vi "cDAQ Open ADC.vi"(8 "error in":errorcluster, 10 "Reset (False)":bool, 11 "cdaq session in":T1={"mclk [Hz]"=12800000.0, "ADC task"="", "mclk reference"="", "fs [Hz]"=50000.0, "queue adc cmd"=refnum, "queue adc data"=refnum, "adc proc ref"=refnum, "channels"=[], "last channels"=[], "timeout"=timestamp(0 s since 1904-01-01), "N"=1000, "mclk mode"=enum."Free running", "ext mclk source"=""} {"last channels"."Channel id" min=0 step=1; "channels"."Channel id" min=0 step=1}) -> (0 "error out":errorcluster, 2 "channel idns":string[](array[string]), 3 "cdaq session out":T1={"mclk [Hz]"=12800000.0, "ADC task"="", "mclk reference"="", "fs [Hz]"=50000.0, "queue adc cmd"=refnum, "queue adc data"=refnum, "adc proc ref"=refnum, "channels"=[], "last channels"=[], "timeout"=timestamp(0 s since 1904-01-01), "N"=1000, "mclk mode"=enum."Free running", "ext mclk source"=""} {"last channels"."Channel id" min=0 step=1; "channels"."Channel id" min=0 step=1})   [LabVIEW 2020]
uses:
  cDAQ Session.ctl
  low_level_old/cdaq_anal_adc_command.ctl
  low_level_old/cdaq_anal_adc_data.ctl
  cDAQ Virtual Channel.ctl
  cDAQ Master Clock Mode.ctl
  <vilib>/Utility/error.llb/Error Cluster From Error Code.vi
  <vilib>/DAQmx/create/channels.llb/DAQmx Create Channel (AI-Voltage-Basic).vi
  <vilib>/DAQmx/configure/timing.llb/DAQmx Timing (Sample Clock).vi
  <vilib>/ErrorRing/Error Ring.xnode
  <resource>/objmgr/daqmx.rc
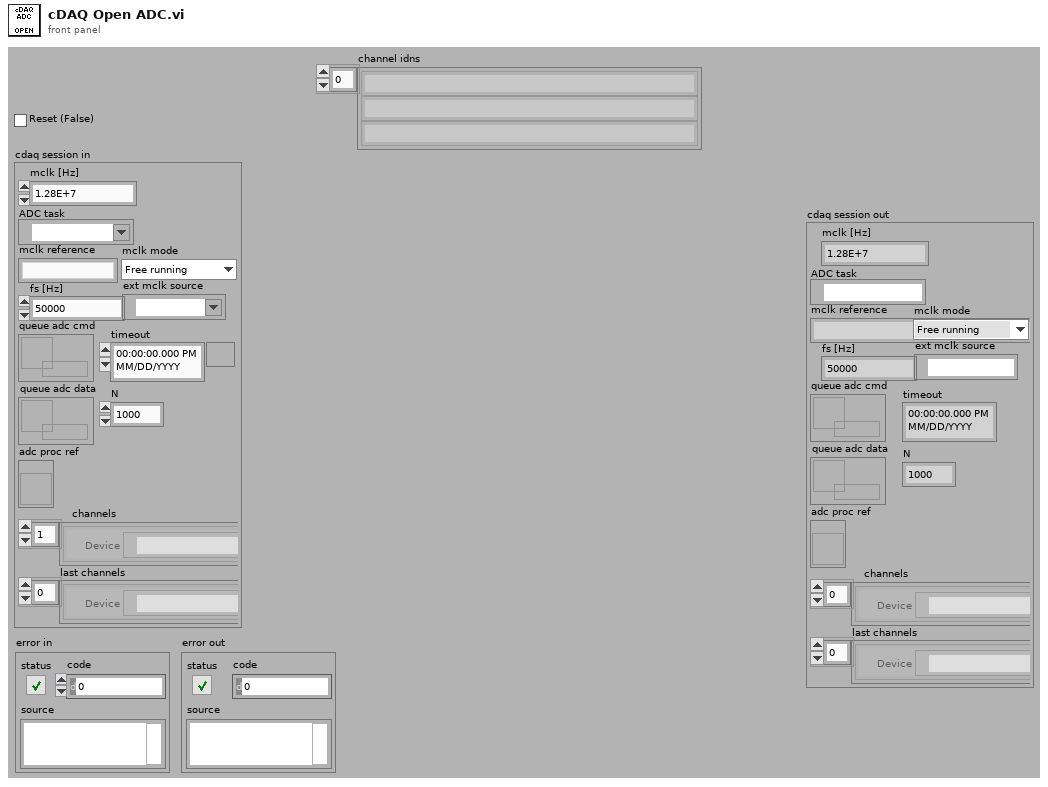
[diagram p1: front panel]
types:
  T1 = typedef "cDAQ Session.ctl" = cluster{"mclk [Hz]":dbl, "ADC task":refnum<k21>, "mclk reference":string, "fs [Hz]":dbl, "queue adc cmd":refnum<queue>, "queue adc data":refnum<queue>, "adc proc ref":refnum<vi>, "channels":T2[], "last channels":T2[], "timeout":timestamp, "N":i32, "mclk mode":T3, "ext mclk source":tag}
  T2 = typedef "cDAQ Virtual Channel.ctl" = cluster{"Device":tag, "Channel id":i32, "btn clr":bool, "btn up":bool, "btn down":bool}
  T3 = typedef "cDAQ Master Clock Mode.ctl" = enum16{"Free running", "Export master clock", "Import master clock"}
  T4 = typedef "cdaq_anal_adc_data.ctl" = cluster{"wave":dbl[][], "timestamp [s]":dbl, "abs timestamp":timestamp, "Aborted":bool}
  T5 = typedef "cdaq_anal_adc_command.ctl" = cluster{"sample to get":i32, "stop":bool, "abort":bool}
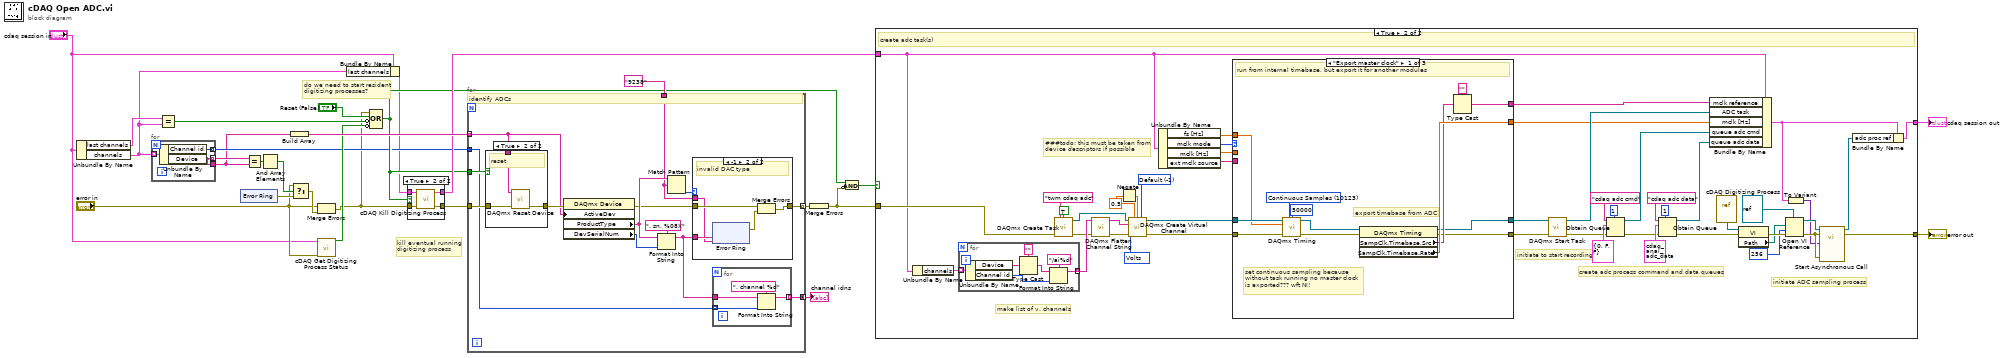
[diagram p0: block diagram]
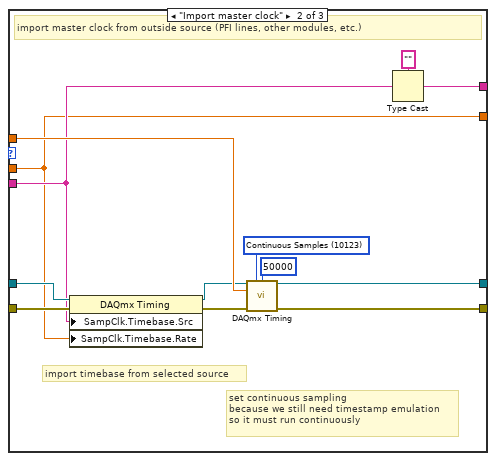
[diagram p4: hidden frame]
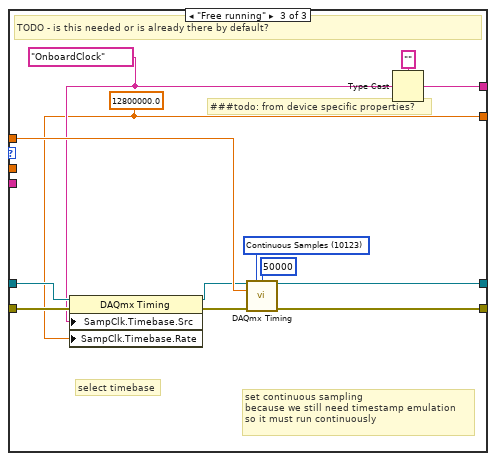
[diagram p5: hidden frame]
diagram:
  # "do we need to start resident\ndigitizing processes?"
  # "kill eventual running\ndigitizing process"
  n1 = Unbundle By Name("cdaq session in") -> ("last channels"=w18:T2[], "channels"=w2:T2[])
  n2 = for {
    tunnel: w2 -> [w30] mode=indexing
    tunnel: [w29] -> w24 mode=indexing
    tunnel: [w29] -> w5
    tunnel: [w28] -> w6 mode=indexing
    n3 = Unbundle By Name(w30) -> ("Channel id"=w28:i32, "Device"=w29:tag)
  }
  n4 = Equal?(x=w18, y=w2) -> (x = y?=w15:bool)
  n5 = xnode "Error Ring"() -> ("error out"=w21:errorcluster)
  n6 = Equal?(x=w24, y=w5) -> (x = y?=w23:bool[])
  n7 = And Array Elements(Boolean array=w23) -> (logical AND=w22:bool)
  n8 = Build Array(w5) -> (w19:tag[])
  n9 = Select(t="error in", s=w22, f=w21) -> (s? t:f=w20:errorcluster)
  n10 = call "cDAQ Get Digitizing Process Status.vi"("error in"="error in", "cdaq session"="cdaq session in") -> ("is running"=w14:bool)  [unwired: 7 in, 2 out]
  n11 = Merge Errors("error in", w20) -> (w4:errorcluster)
  n12 = Bundle By Name(cluster="cdaq session in", "last channels"=w2) -> (w3:T1)
  n13 = Compound Arithmetic op=OR(w4, "Reset (False)", invert w15, invert w14) -> (w9:bool)
  n14 = case shown="True" w9 {
    tunnel: w4 -> [w32 w36]
    tunnel: [w32 w35] -> w11
    tunnel: w3 -> [w31 w34]
    tunnel: [w31 w33] -> w10
    frame False {
    }
    frame True {
      n15 = call "cDAQ Kill Digitizing Process.vi"("error in"=w36, "cdaq session in"=w34) -> ("error out"=w35:errorcluster, "cdaq session out"=w33:T1)  [unwired: 8 in]
    }
  }
  n16 = for {
    tunnel: w19 -> [w49] mode=indexing
    tunnel: w11 -> [w43]
    tunnel: "9238" -> [w41]
    tunnel: [w42] -> w27 mode=indexing
    tunnel: w9 -> [w40]
    tunnel: w6 -> [w38]
    tunnel: [w37] -> w12 mode=concatenating
    # "identify ADCs"
    n17 = case shown="True" w40 {
      tunnel: [w55 w58] -> w50
      tunnel: w49 -> [_ w57]
      tunnel: w43 -> [w55 w56]
      frame False {
      }
      frame True {
        # "reset"
        n18 = call <vilib>:"DAQmx Reset Device.vi"("device in"=w57, "error in"=w56) -> ("error out"=w58:errorcluster)  [unwired: 13 in]
      }
    }
    n19 = property class="DAQmx Device"(error in=w50, "ActiveDev"=w49) -> (error out=w44:errorcluster, "ProductType"=w46:string, "DevSerialNum"=w48:u32)  [unwired: 1 in, 1 out]
    n20 = Format Into String(format string=", sn. %08X", initial string=w46, w48) -> (resulting string=w39:string)  [unwired: 1 in, 1 out]
    n21 = Match Pattern(string=w46, regular expression=w41) -> (offset past match=w45:i32)  [unwired: 1 in, 3 out]
    n22 = case shown="-1" w45 {
      tunnel: w44 -> [w59 w64]
      tunnel: w39 -> [_ w61]
      tunnel: [w59 w62] -> w42
      tunnel: w41 -> [_ w60]
      frame Default {
      }
      frame -1 {
        # "invalid DAC type"
        n23 = xnode "Error Ring"("parameter 0"=w61, "parameter 1"=w60) -> ("error out"=w63:errorcluster)
        n24 = Merge Errors(w64, w63) -> (w62:errorcluster)
      }
    }
    n25 = for {
      tunnel: w39 -> [w54]
      tunnel: w38 -> [w52] mode=indexing
      tunnel: [w51] -> w37 mode=indexing
      n26 = Format Into String(format string=", channel %d", initial string=w54, w52) -> (resulting string=w51:string)  [unwired: 1 in, 1 out]
    }
  }
  "channel idns" <- w12
  n27 = Merge Errors(w27) -> (w7:errorcluster)
  n28 = Compound Arithmetic op=AND(w9, invert w7) -> (w8:bool)
  n29 = case shown="True" w8 {
    tunnel: w10 -> [w74 w87]
    tunnel: [w73 w92] -> w26
    tunnel: [w74 w89] -> w25
    tunnel: w7 -> [w73 w88]
    frame False {
    }
    frame True {
      w113 = 0.5 ("maximum value")
      w122 = -1 items=["Default"=-1, "RSE"=10083, "Differential"=10106, "Pseudodifferential"=12529] ("output terminal configuration")
      w120 = 10348 items=["Volts"=10348, "From Custom Scale"=10065] ("units")
      # "###todo: this must be taken from\ndevice descriptors if possible"
      # "make list of v. channels"
      # "initiate ADC sampling process"
      # "create adc process command and data queues"
      # "initiate to start recording"
      # "create adc task(s)"
      n30 = Unbundle By Name(w87) -> ("channels"=w86:T2[])
      n31 = for {
        tunnel: [w167] -> w118 mode=indexing
        tunnel: w86 -> [w166] mode=indexing
        n32 = Unbundle By Name(w166) -> ("Device"=w164:tag, "Channel id"=w162:i32)
        n33 = Type Cast(type="", x=w164) -> (*(type *) &x=w163:string)
        n34 = Format Into String(format string="/ai%d", initial string=w163, w162) -> (resulting string=w167:string)  [unwired: 1 in, 1 out]
      }
      n35 = call <vilib>:"DAQmx Create Task.vi"("new task name"="twm cdaq adc", "auto cleanup"=TRUE, "error in"=w88) -> ("task out"=w115:refnum<k21>, "error out"=w116:errorcluster)  [unwired: 11 in]
      n36 = call <vilib>:"DAQmx Flatten Channel String.vi"("names in"=w118, "error in"=w116) -> ("names out"=w119:string, "error out"=w117:errorcluster)  [unwired: 12 in]
      n37 = Negate(x=w113) -> (-x=w112:dbl)
      n38 = call-poly <vilib>:"DAQmx Create Virtual Channel.vi"("task in"=w115, "maximum value"=w113, "minimum value"=w112, "input terminal configuration"=w122, "physical channels"=w119, "units"=w120, "error in"=w117) -> ("task out"=w83:refnum<k21>, "error out"=w84:errorcluster)  [unwired: 7 in]
      n39 = Unbundle By Name(w87) -> ("fs [Hz]"=w79:dbl, "mclk mode"=w80:T3, "mclk [Hz]"=w78:dbl, "ext mclk source"=w76:tag)
      n40 = case shown="\"Export master clock\"" w80 {
        tunnel: [w135 w138 w151] -> w75
        tunnel: w84 -> [w132 w145 w158]
        tunnel: w83 -> [w131 w142 w155]
        tunnel: w79 -> [w125 w146 w159]
        tunnel: [w126 w140 w153] -> w77
        tunnel: [w124 w137 w149] -> w82
        tunnel: w78 -> [_ w138 _]
        tunnel: w76 -> [_ w139 _]
        tunnel: [w123 w136 w150] -> w81
        frame "Export master clock" {
          w134 = 10123 items=["Finite Samples"=10178, "Continuous Samples"=10123, "Hardware Timed Single Point"=12522] ("sample mode")
          # "set continuous sampling because\nwithout task running no master clock \nis exported??? wft NI!"
          # "export timebase from ADC"
          # "run from internal timebase, but export it for another modules"
          n41 = call-poly <vilib>:"DAQmx Timing.vi"("task/channels in"=w131, "sample mode"=w134, "samples per channel"=50000, "rate"=w125, "error in"=w132) -> ("task out"=w129:refnum<k21>, "error out"=w130:errorcluster)  [unwired: 9 in]
          n42 = property class="DAQmx Timing"(reference=w129, error in=w130) -> (reference out=w123:refnum<k21>, error out=w124:errorcluster, "SampClk.Timebase.Src"=w127:tag, "SampClk.Timebase.Rate"=w135:dbl)
          n43 = Type Cast(type="", x=w127) -> (*(type *) &x=w126:string)
        }
        frame "Import master clock" {
          w148 = 10123 items=["Finite Samples"=10178, "Continuous Samples"=10123, "Hardware Timed Single Point"=12522] ("sample mode")
          # "set continuous sampling\nbecause we still need timestamp emulation\nso it must run continuously"
          # "import timebase from selected source"
          # "import master clock from outside source (PFI lines, other modules, etc.)"
          n44 = property class="DAQmx Timing"(reference=w142, error in=w145, "SampClk.Timebase.Src"=w139, "SampClk.Timebase.Rate"=w138) -> (reference out=w143:refnum<k21>, error out=w144:errorcluster)
          n45 = call-poly <vilib>:"DAQmx Timing.vi"("task/channels in"=w143, "sample mode"=w148, "samples per channel"=50000, "rate"=w146, "error in"=w144) -> ("task out"=w136:refnum<k21>, "error out"=w137:errorcluster)  [unwired: 9 in]
          n46 = Type Cast(type="", x=w139) -> (*(type *) &x=w140:string)
        }
        frame "Free running" {
          w151 = 12800000.0 ("SampClk.Timebase.Rate")
          w152 = tag "OnboardClock" ("SampClk.Timebase.Src")
          w161 = 10123 items=["Finite Samples"=10178, "Continuous Samples"=10123, "Hardware Timed Single Point"=12522] ("sample mode")
          # "###todo: from device specific properties?"
          # "set continuous sampling\nbecause we still need timestamp emulation\nso it must run continuously"
          # "select timebase"
          # "TODO - is this needed or is already there by default?"
          n47 = property class="DAQmx Timing"(reference=w155, error in=w158, "SampClk.Timebase.Src"=w152, "SampClk.Timebase.Rate"=w151) -> (reference out=w156:refnum<k21>, error out=w157:errorcluster)
          n48 = call-poly <vilib>:"DAQmx Timing.vi"("task/channels in"=w156, "sample mode"=w161, "samples per channel"=50000, "rate"=w159, "error in"=w157) -> ("task out"=w150:refnum<k21>, "error out"=w149:errorcluster)  [unwired: 9 in]
          n49 = Type Cast(type="", x=w152) -> (*(type *) &x=w153:string)
        }
      }
      n50 = call <vilib>:"DAQmx Start Task.vi"("task/channels in"=w81, "error in"=w82) -> ("task out"=w102:refnum<k21>, "error out"=w85:errorcluster)  [unwired: 12 in]
      n51 = Obtain Queue(max queue size (-1, unlimited)=1, name (unnamed)="cdaq adc cmd", element data type=T5 {"sample to get"=0, "stop"=FALSE, "abort"=FALSE} ("adc cmd"), error in (no error)=w85) -> (queue out=w104:refnum<queue>, error out=w105:errorcluster)  [unwired: 1 in, 1 out]
      n52 = Obtain Queue(max queue size (-1, unlimited)=1, name (unnamed)="cdaq adc data", element data type=T4 {"wave"=[], "timestamp [s]"=0.0, "abs timestamp"=timestamp(0 s since 1904-01-01), "Aborted"=FALSE} ("adc data"), error in (no error)=w105) -> (queue out=w103:refnum<queue>, error out=w93:errorcluster)  [unwired: 1 in, 1 out]
      n53 = Bundle By Name(cluster=w87, "mclk reference"=w77, "ADC task"=w102, "mclk [Hz]"=w75, "queue adc cmd"=w104, "queue adc data"=w103) -> (w91:T1)
      n54 = vi-ref "cDAQ Digitizing Process.vi"() -> (w100:refnum<vi>)
      n55 = property class="VI"(reference=w100, error in=w93) -> (error out=w99:errorcluster, "Path"=w97:path)  [unwired: 1 out]
      n56 = Open VI Reference(type specifier VI Refnum (for type only)=refnum<vi> refnum, vi path=w97, options=256, error in (no error)=w99) -> (vi reference=w101:refnum<vi>, error out=w98:errorcluster)  [unwired: 2 in]
      n57 = To Variant(anything=w91) -> (Variant=w94:variant)
      n58 = call-by-ref "Start Asynchronous Call"(reference=w101, error in=w98, "error in"=w98, "cdaq session"=w94) -> (reference out=w90:refnum<vi>, error out=w92:errorcluster)  [unwired: 9 in, 1 out]
      n59 = Bundle By Name(cluster=w91, "adc proc ref"=w90) -> (w89:T1)
    }
  }
  "cdaq session out" <- w25
  "error out" <- w26
